vi "Add object to group.vi"(8 "error in (no error)":errorcluster, 10 "system object":refnum<class "system object.lvclass">, 11 "Folder in":refnum<class "Folder.lvclass">) -> (0 "error out":errorcluster, 3 "Folder out":refnum<class "Folder.lvclass">)   [LabVIEW 2020, in "Folder.lvclass"]
uses:
  Folder.lvclass
  C:/PA_Source/advent-of-code/2022/Paul/07/classes/system object/system object.lvclass
  system object/system object.lvclass
  Folder.lvclass/Folder.ctl
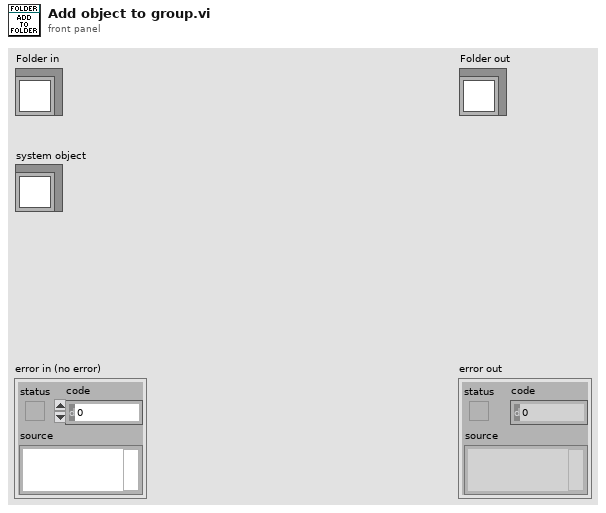
[diagram p1: front panel]
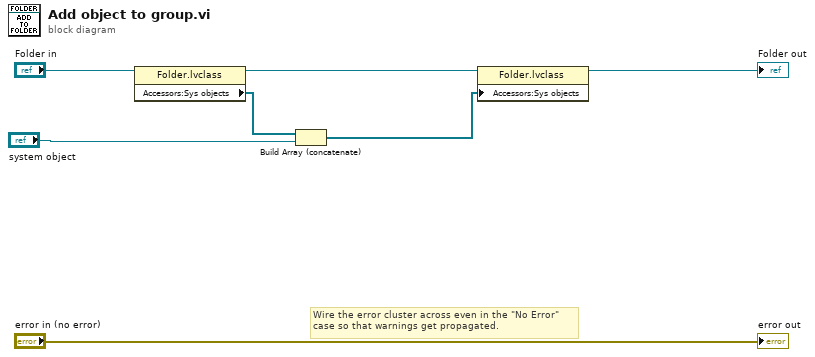
[diagram p0: block diagram]
diagram:
  # "Wire the error cluster across even in the \"No Error\"\ncase so that warnings get propagated."
  n1 = property class="Folder.lvclass"(reference="Folder in") -> (reference out=w4:refnum<class "Folder.lvclass">, "Accessors:Sys objects"=w2:refnum<class "system object.lvclass">[])  [unwired: 1 in, 1 out]
  n2 = Build Array (concatenate)(w2, "system object") -> (w1:refnum<class "system object.lvclass">[])
  n3 = property class="Folder.lvclass"(reference=w4, "Accessors:Sys objects"=w1) -> (reference out=→"Folder out":refnum<class "Folder.lvclass">)  [unwired: 1 in, 1 out]
  "error out" <- "error in (no error)"
